vi "Write Port.vi"(2 "Timeout":i16, 8 "error in (no error)":errorcluster, 9 "Port":T1="Mod6\\Port1", 10 "Data":u8, 11 "TestMPU in":refnum<class "TestMPU.lvclass">) -> (0 "error out":errorcluster, 1 "Timeouted":bool, 3 "TestMPU out":refnum<class "TestMPU.lvclass">)   [LabVIEW 2018, in "TestMPU.lvclass"]
uses:
  TestMPU.lvclass
  src/PortType.ctl
  TestMPU.lvclass/TestMPU.ctl
  <vilib>/rvi/DataTransferAndStorage/Container/Common/niFpgaContainerExecOnDevCompGetState.vi
  <vilib>/rvi/Emulation/niFpgaEmulationIsFPGAContextNoSignature.vi
  <vilib>/rvi/Emulation/niFpgaSctlEmulationGetInTimedLoop.vi
  <vilib>/rvi/errors/niFpgaSetErrorForExecOnDevCompSimple.vi
  <vilib>/rvi/eio/common/nirviEmuReportErrorAndStop.vi
  <vilib>/rvi/DataTransferAndStorage/Container/Common/niFpgaContainerGetUniqueNameForEmu.vi
  <vilib>/rvi/FIFO/Fifo_Resource/nirvififoEmulationSetSize.vi
  <vilib>/rvi/FIFO/Fifo_Resource/nirviFifoEmulationQueueMgr.vi
  <instcachedir>/0/nirviFifoEmulationQueueMgr_E5CAEC123FF24DC58D834DCA3CDAA9B5.lvgen/nirviFifoEmulationQueueMgr_E5CAEC123FF24DC58D834DCA3CDAA9B5_001.vi
  <vilib>/rvi/FIFO/Fifo_Resource/nirvififoEmulationDetermineInputValidOut.vi
  <vilib>/rvi/FIFO/Fifo_Resource/nirvififoEmulationCreateLock.vi
  <vilib>/rvi/Emulation/niFpgaProcessEmulError.vi
  <vilib>/rvi/FIFO/Fifo_Resource/nirvififoEmulationObtainLock.vi
  <vilib>/rvi/FIFO/Fifo_Resource/nirvififoEmulationReleaseLock.vi
  <vilib>/rvi/occurrence/nirviWaitOnOccurrenceBase.vi
  <vilib>/rvi/errors/nirviReportUnexpectedCaseInternalError.vi
  <vilib>/rvi/errors/nirviReportUnexpectedCaseInternalError (U32).vi
  <vilib>/Utility/error.llb/Clear Errors.vi
  <vilib>/rvi/interface/RandomDataEmulation/niFpgaRandomDataHandleErrors.vi
  <vilib>/rvi/DataTransferAndStorage/Container/XNode/niFpgaContainer.xnode
  <vilib>/rvi/FIFO/Fifo_Resource/niFpgaFifoEmulationRefIn.vi
  src/MPU.lvclass
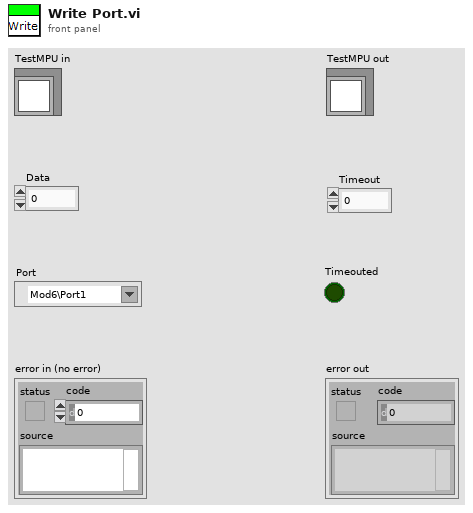
[diagram p1: front panel]
types:
  T1 = typedef "PortType.ctl" = refnum<k21>
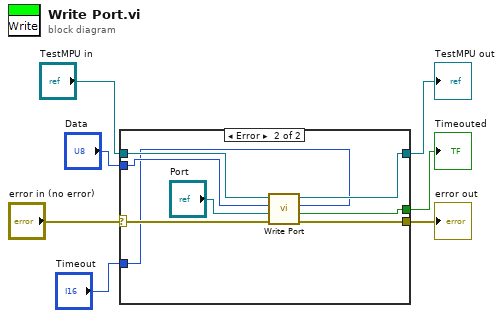
[diagram p0: block diagram]
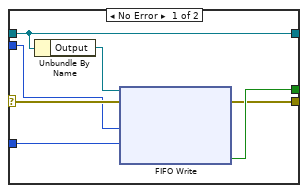
[diagram p2: hidden frame]
diagram:
  n1 = case shown="Error" "error in (no error)" {
    selector: "error in (no error)" -> [w13 w17]
    tunnel: [w9 w22] -> w7
    tunnel: [w10 w21] -> w6
    tunnel: [w8 w20] -> w5
    tunnel: "Timeout" -> [w11 w16]
    tunnel: "Data" -> [w12 w19]
    tunnel: "TestMPU in" -> [w8 w18]
    frame No Error {
      n2 = Unbundle By Name(w8) -> ("Output"=w14:refnum<k21>)
      n3 = xnode "FIFO Write"("Element"=w12, "Timeout"=w11, "error in (no error)"=w13, "FIFO In"=w14) -> ("Timed Out?"=w10:bool, "error out"=w9:errorcluster)  [unwired: 1 out]
    }
    frame Error {
      n4 = call-parent "Write Port.vi"("Timeout"=w16, "error in (no error)"=w17, "Port"="Port", "Data"=w19, "MPU in"=w18) -> ("error out"=w22:errorcluster, "Timeouted"=w21:bool, "MPU out"=w20:refnum<class "TestMPU.lvclass">)  [unwired: 4 in]
    }
  }
  "error out" <- w7
  "TestMPU out" <- w5
  "Timeouted" <- w6
